vi "关闭工作簿集.vi"(8 "错误输入（无错误）":errorcluster, 11 "工作薄引用":refnum<k7>) -> (0 "错误输出":errorcluster, 3 "工作薄引用输出":refnum<k7>)   [LabVIEW 2013, in "excel处理.lvlib"]
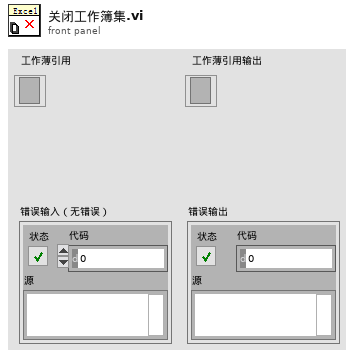
[diagram p1: front panel]
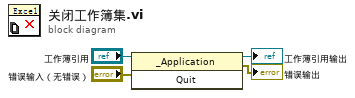
[diagram p0: block diagram]
diagram:
  n1 = invoke on="调用节点" class="_Application" method="Quit"(reference="工作薄引用", error in="错误输入（无错误）") -> (reference out=→"工作薄引用输出":refnum<k7>, error out=→"错误输出":errorcluster)  [unwired: 1 in, 1 out]
